vi "FIFO Bucket.vi"() -> ()   [LabVIEW 2010]
doc: "This VI demonstrates how elements are written to and read from a Target-Scoped FIFO on FPGA. When the user selects write, elements will be written to the FIFO in increasing order. If the FIFO runs out of room to write the data, the FIFO Full LED will become true. When the user selects to read from the FIFO, a different loop will begin to read from the FIFO one element at a time and the element will be displayed in the Element Read indicator. If the FIFO runs out of elements to read, the FIFO Empty LED will become true. The bucket is used to keep track of how many elements are currently in the FIFO. This number is calculated by taking the number of successful writes to the FIFO and subtracting the number of successful reads."
uses:
  <vilib>/rvi/DataTransferAndStorage/Container/XNode/niFpgaContainer.xnode
  <vilib>/rvi/FIFO/Fifo_Resource/nirvififoEmulationSetSize.vi
  <vilib>/rvi/DataTransferAndStorage/Container/Common/niFpgaContainerGetUniqueNameForEmu.vi
panel:
  out "Element Read":u16
  out "FIFO Empty":bool
  out "FIFO Full":bool
  out "Bucket":u16(slide) scale=0.0..36.0
  in  "Read":bool
  in  "Write":bool
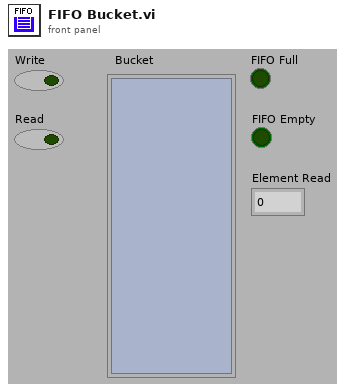
[diagram p1: front panel]
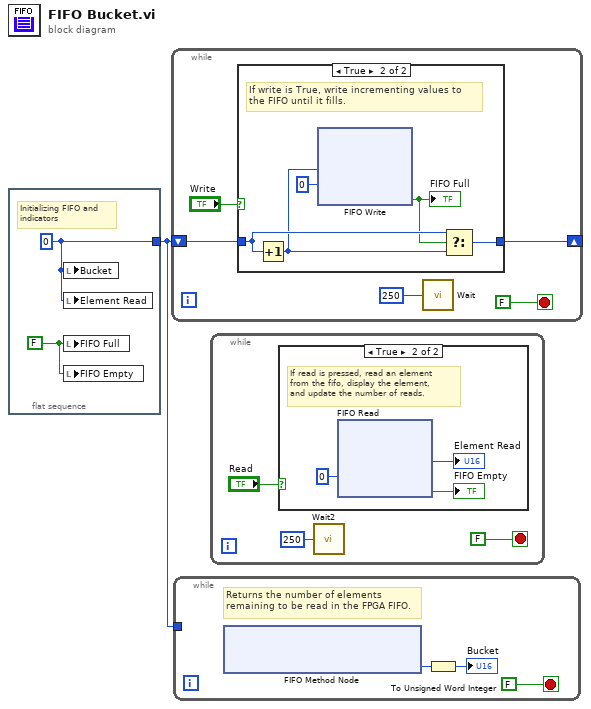
[diagram p0: block diagram]
diagram:
  n1 = flat-sequence {
    tunnel: [w2] -> w1
    frame #0 {
      w3 = FALSE ("FIFO Full")
      w2 = u16 0 ("writes")
      # "Initializing FIFO and\nindicators"
      n2 = local write "Bucket"(w2) -> ()
      n3 = local write "Element Read"(w2) -> ()
      n4 = local write "FIFO Full"(w3) -> ()
      n5 = local write "FIFO Empty"(w3) -> ()
    }
  }
  n6 = while {
    shift-right: [w4] -> _
    shift-left: w1 -> [w7]
    stop <- FALSE stop-if-true
    n7 = case shown="True" "Write" {
      tunnel: w7 -> [w9 w13]
      tunnel: [w9 w14] -> w4
      frame False {
        # "If write is False, do not write to the FIFO"
      }
      frame True {
        # "If write is True, write incrementing values to the FIFO until it fills."
        n8 = Increment(x=w13) -> (x+1=w12:u16)
        n9 = xnode ("FIFO Write")("Element"=w12, "Timeout"=0) -> ("Timed Out?"=w10:bool)  [unwired: 1 in, 1 out]
        "FIFO Full" <- w10
        n10 = Select(t=w13, s=w10, f=w12) -> (s? t:f=w14:u16)
      }
    }
    n11 = call "Wait"("Count(mSec)"=u32 250) -> ()  [unwired: 1 out]
  }
  n12 = while {
    tunnel: w1 -> [_]
    stop <- FALSE stop-if-true
    # "Returns the number of elements remaining to be read in the FPGA FIFO."
    n13 = xnode ("FIFO Method Node")() -> ("Number of Elements to Read"=w67:u32)  [unwired: 1 in, 1 out]
    n14 = To Unsigned Word Integer(number=w67) -> (unsigned 16bit integer=→"Bucket":u16)
  }
  n15 = while {
    stop <- FALSE stop-if-true
    n16 = case shown="True" "Read" {
      frame False {
        # "If read False, do not \nread from the FIFO."
      }
      frame True {
        # "If read is pressed, read an element\nfrom the fifo, display the element,\nand update the number of reads."
        n17 = xnode ("FIFO Read")("Timeout"=0) -> ("Element"=→"Element Read":u16, "Timed Out?"=→"FIFO Empty":bool)  [unwired: 1 in, 1 out]
      }
    }
    n18 = call "Wait2"("Count(mSec)"=u32 250) -> ()  [unwired: 1 out]
  }
